vi "CHD_SIM_MOTOR_ALLOC.vi"(11 "Index":i32) -> ()   [LabVIEW 2019]
uses:
  CHD_SIM_SIM_Globals.vi
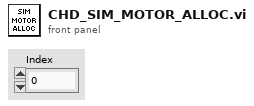
[diagram p1: front panel]
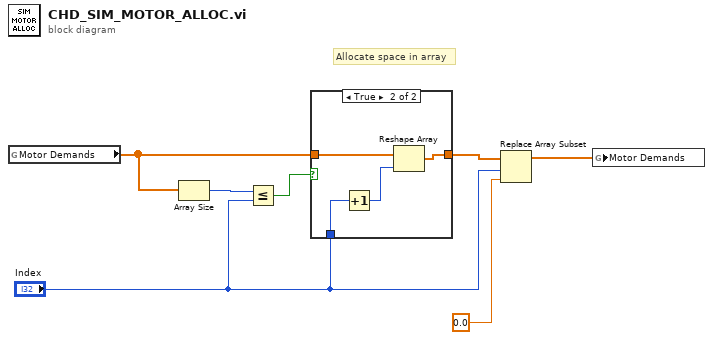
[diagram p0: block diagram]
diagram:
  # "Allocate space in array"
  n1 = global read "CHD_SIM_SIM_Globals.vi" "Motor Demands"() -> (w5:dbl[])
  n2 = Array Size(array=w5) -> (size(s)=w4:i32)
  n3 = Less Or Equal?(x=w4, y="Index") -> (x <= y?=w2:bool)
  n4 = case shown="True" w2 {
    tunnel: [w8 w12] -> w7
    tunnel: w5 -> [w8 w11]
    tunnel: "Index" -> [_ w9]
    frame False {
    }
    frame True {
      n5 = Increment(x=w9) -> (x+1=w10:i32)
      n6 = Reshape Array(w11, w10) -> (w12:dbl[])
    }
  }
  n7 = Replace Array Subset(array=w7, new element=0.0 ("new element/subarray"), index="Index") -> (w6:dbl[])
  n8 = global write "CHD_SIM_SIM_Globals.vi" "Motor Demands"(w6) -> ()
